vi "open.vi"(0 "TCSettings in":refnum<class "TCSettings.lvclass">, 11 "error in (no error)":errorcluster) -> (4 "TCSettings out":refnum<class "TCSettings.lvclass">, 6 "SelectedSet":string, 8 "SelectedVersion":string, 10 "Canceled":bool, 15 "error out":errorcluster)   [LabVIEW 2016, in "Settings.lvlib" / "TCSettings.lvclass"]
uses:
  TCSettings.lvclass
  C:/Users/aanania/Documents/ts_monochromator_windows/MonoSettings/Settings/Settings/Setting.lvclass
  Settings/Setting.lvclass/Setting.ctl
  Settings/Setting.lvclass
panel:
  in  "Create New":bool
  in  "Cancel":bool
  in  "Edit Selected":bool
  in  "Available Settings":i32(listbox)
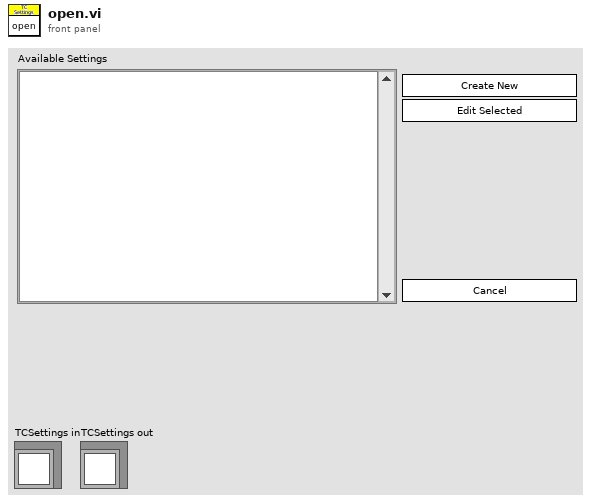
[diagram p1: front panel]
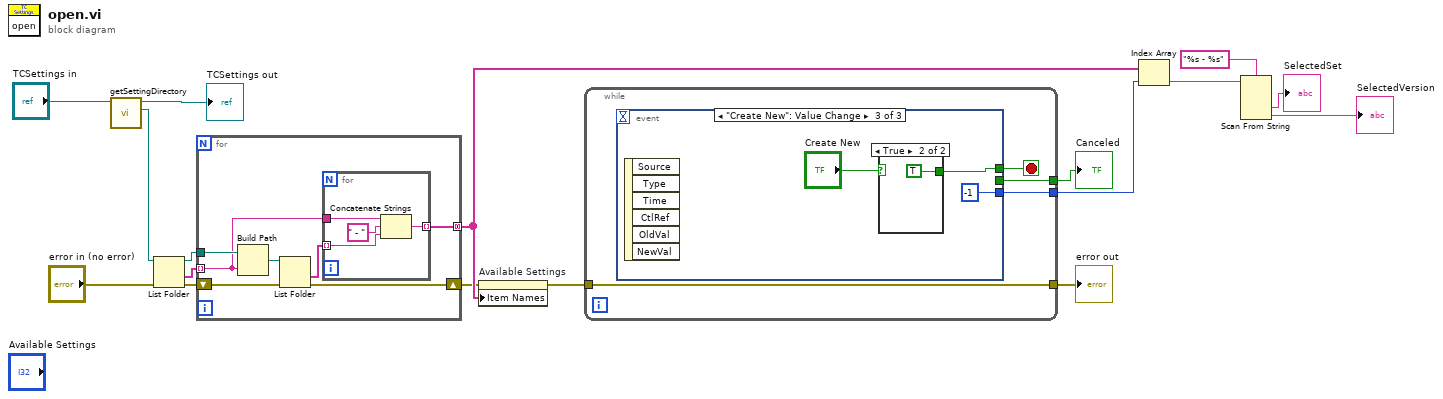
[diagram p0: block diagram]
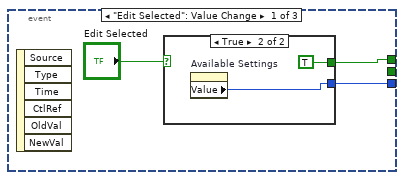
[diagram p2: hidden frame]
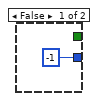
[diagram p3: hidden frame]
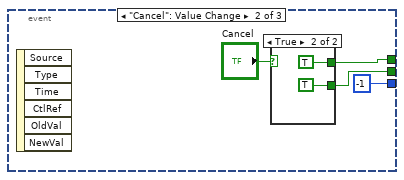
[diagram p4: hidden frame]
diagram:
  n1 = call "getSettingDirectory.vi"("BaseSetting in"="TCSettings in") -> ("SettingDirectory"=w13:path, "BaseSetting out"=→"TCSettings out":refnum<class "TCSettings.lvclass">)  [unwired: 9 in]
  n2 = List Folder(path=w13, error in="error in (no error)") -> (path out=w11:path, folder names=w12:string[], error out=w8:errorcluster)  [unwired: 2 in, 1 out]
  n3 = for {
    tunnel: w12 -> [w21] mode=indexing
    tunnel: w11 -> [w24]
    tunnel: [w20] -> w10 mode=concatenating
    shift-right: [w18] -> w7
    shift-left: w8 -> [w19]
    n4 = Build Path(base path=w24, name or relative path=w21) -> (appended path=w23:path)
    n5 = List Folder(path=w23, error in=w19) -> (folder names=w22:string[], error out=w18:errorcluster)  [unwired: 2 in, 2 out]
    n6 = for {
      tunnel: w22 -> [w27] mode=indexing
      tunnel: w21 -> [w28]
      tunnel: [w25] -> w20 mode=indexing
      n7 = Concatenate Strings(w28, " - " ("string"), w27) -> (w25:string)
    }
  }
  n8 = property on="Available Settings" class="LstBox (strict)"(error in=w7, "Item Names"=w10) -> (error out=w15:errorcluster)  [unwired: 1 in, 1 out]
  n9 = while {
    tunnel: [w31] -> w14
    tunnel: [w30] -> w17
    tunnel: [w29] -> w16
    tunnel: w15 -> [w29]
    stop <- w32 stop-if-true
    n10 = event shown="[2] \"Create New\": Value Change" {
      selector: _ -> [_ _ _]
      dyn-events: _ -> [_ _ _]
      timeout: _ -> [_ _ _]
      tunnel: [w34 w41 w45] -> w32
      tunnel: [_ w40 _] -> w31
      tunnel: [w33 -1 ("Value") -1 ("Value")] -> w30
      event "Edit Selected": Value Change {
        n11 = event-data() -> ()  [unwired: 1 in, 6 out]
        n12 = case shown="True" "Edit Selected" {
          tunnel: [_ TRUE] -> w34
          tunnel: [-1 ("Value") w37] -> w33
          frame False {
          }
          frame True {
            n13 = property on="Available Settings" class="LstBox (strict)"() -> ("Value"=w37:i32)  [unwired: 2 in, 2 out]
          }
        }
      }
      event "Cancel": Value Change {
        n14 = event-data() -> ()  [unwired: 1 in, 6 out]
        n15 = case shown="True" "Cancel" {
          tunnel: [_ TRUE] -> w41
          tunnel: [_ TRUE] -> w40
          frame False {
          }
          frame True {
          }
        }
      }
      event "Create New": Value Change {
        n16 = event-data() -> ()  [unwired: 1 in, 6 out]
        n17 = case shown="True" "Create New" {
          tunnel: [_ TRUE] -> w45
          frame False {
          }
          frame True {
          }
        }
      }
    }
  }
  "error out" <- w16
  "Canceled" <- w14
  n18 = Index Array(array=w10, index=w17) -> (element=w5:string)
  n19 = Scan From String(format string="%s - %s", input string=w5) -> (output 1=→"SelectedSet":string, output 2=→"SelectedVersion":string)  [unwired: 4 in, 3 out]
